vi "NIFPGA-MCS.initialize.vi"(0 "i ref in":refnum<vi>, 3 "ms timeout (10000)":i32=10000, 5 "error in (no error)":errorcluster) -> (14 "i ref out":refnum<vi>, 17 "timed out":bool, 19 "error out":errorcluster)   [LabVIEW 2014, in "NIFPGA-MCS.lvlib"]
doc: "Initializes the MCS."
uses:
  NIFPGA-MCS.lvlib
  instr.lib/NI-FPGA-MCS/host/instrumentDriver/NI-FPGA-MCS_Driver.lvlib
  CS_Core/CSApplicationBaseClasses/DeviceBase/DeviceBase.lvlib
  CSlibraries/UtilityLib/UtilityLib.lvlib
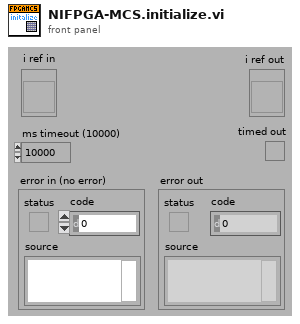
[diagram p1: front panel]
types:
  T1 = typedef "NIFPGA-MCS.lvlib/NIFPGA-MCS.i attribute.ctl" = cluster{"fpgaViRef":T2}
  T2 = typedef "NI-FPGA-MCS_Driver.lvlib/fpga_vi_ref.ctl" = refnum<k20>
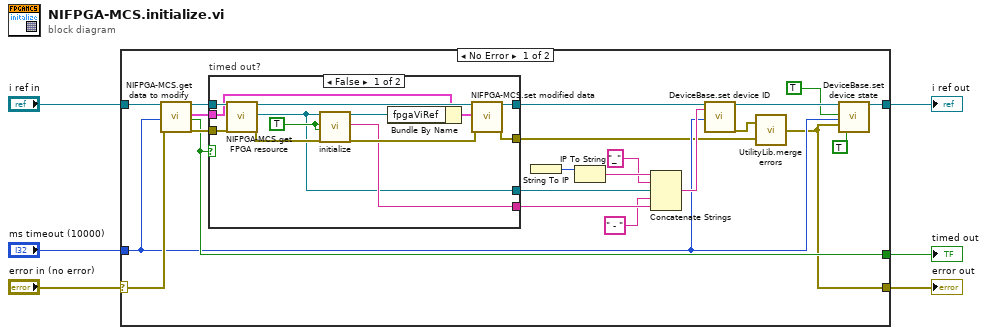
[diagram p0: block diagram]
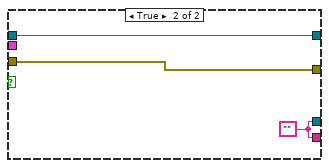
[diagram p2: hidden frame]
diagram:
  n1 = case shown="No Error" "error in (no error)" {
    selector: "error in (no error)" -> [w27 w45]
    tunnel: "i ref in" -> [w28 w46]
    tunnel: [w18 w46] -> w4
    tunnel: [w12 w45] -> w3
    tunnel: "ms timeout (10000)" -> [w17 _]
    tunnel: [w20 _] -> w1
    frame No Error {
      n2 = call "NIFPGA-MCS.get data to modify.vi"("i ref in"=w28, "ms timeout (10000)"=w17, "error in (no error)"=w27) -> ("i ref out"=w26:refnum<vi>, "i attribute"=w24:T1, "timed out"=w20:bool, "error out"=w25:errorcluster)  [unwired: 13 in]
      n3 = case "timed out?" shown="False" w20 {
        tunnel: w26 -> [w40 w44]
        tunnel: w25 -> [w39 w43]
        tunnel: w24 -> [w36 _]
        tunnel: [w33 w44] -> w23
        tunnel: [w29 w42] -> w22
        tunnel: [w31 w42] -> w11
        tunnel: [w30 w43] -> w13
        frame False {
          w32 = TRUE ("idQuery (False)")
          n4 = call "NIFPGA-MCS.get FPGA resource.vi"("i ref in"=w40, "error in (no error)"=w39) -> ("i ref out"=w38:refnum<vi>, "resourceName"=w29:refnum<visa-resource-name>, "error out"=w41:errorcluster)  [unwired: 15 in]
          n5 = call "initialize.vi"("resourceName"=w29, "idQuery (False)"=w32, "reset (True)"=w32, "error in (no error)"=w41) -> ("fpgaViRef"=w35:T2, "instrumentFirmwareRevision"=w31:string, "error out"=w37:errorcluster)  [unwired: 13 in]
          n6 = Bundle By Name(cluster=w36, "fpgaViRef"=w35) -> (w34:T1)
          n7 = call "NIFPGA-MCS.set modified data.vi"("i ref in"=w38, "i attribute"=w34, "error in (no error)"=w37) -> ("i ref out"=w33:refnum<vi>, "error out"=w30:errorcluster)  [unwired: 15 in]
        }
        frame True {
          w42 = "" ("instrumentFirmwareRevision")
        }
      }
      n8 = String To IP() -> (0:w9:u32)  [unwired: 1 in]
      n9 = IP To String(2:w9) -> (0:w8:string)  [unwired: 1 in]
      n10 = Concatenate Strings(w8, "_" ("string"), w22, " - " ("string"), w11) -> (w21:string)
      n11 = call "DeviceBase.set device ID.vi"("i ref in"=w23, "deviceID"=w21, "ms timeout (10000)"=w17) -> ("i ref out"=w19:refnum<vi>, "error out"=w14:errorcluster)  [unwired: 14 in, 1 out]
      n12 = call "UtilityLib.merge errors.vi"("error2 (no error)"=w13, "error1 (no error)"=w14) -> ("error out"=w12:errorcluster)
      n13 = call "DeviceBase.set device state.vi"("i ref in"=w19, "implicit"=TRUE, "ms timeout (10000)"=w17, "device error"=w12, "mayResetError (FALSE)"=TRUE) -> ("i ref out"=w18:refnum<vi>)  [unwired: 12 in, 2 out]
    }
    frame Error {
    }
  }
  "error out" <- w3
  "i ref out" <- w4
  "timed out" <- w1
